vi "Vision_Left_R2.0_startup_test.vi"() -> ()   [LabVIEW 2015]
uses:
  <vilib>/vision/Pattern Matching.llb/IMAQ Curve Parameters.ctl
  <vilib>/vision/Pattern Matching.llb/IMAQ Match Range Setting.ctl
panel:
  in  "Sub - 2 File Path 2******":path=path "/home/lvuser/natinst/bin/BeaconTemplates/2_beacons_right.png"
  out "New Min Score":dbl=879.6385864257812
  out "New Low Scale":dbl=38.665856552124026
  out "New high Scale":dbl=79.77148170471192
  in  "Absolute\nMinimum Score":dbl=800.0
  in  "Absolute\nMaximum Scale":dbl=300.0
  in  "Absolute\nMinimum Scale":dbl=10.0
  in  "Score Decay \nFactor":dbl=50.0
  in  "ROI_factor(Horiztonal) (4 b)":sgl=5.0
  in  "ROI_factor(vertical) (4 b)":sgl=1.5
  in  "ROI_factor(vertical) (5 b)":sgl=2.7
  in  "ROI_factor(Horiztonal) (5 b)":sgl=4.7
  in  "ROI_factor(Horiztonal) (2 b)":sgl=1.5
  in  "ROI_factor(vertical) (2 b)":sgl=2.5
  in  "Minimum Score\nSub 2":dbl=950.0
  in  "Minimum Score\nSub 3":dbl=900.0
  in  "Minimum Score\nSub 4":dbl=850.0
  in  "Minimum Score\nNormal 5":dbl=800.0
  in  "ROBOT STATE\n(fwd, bwd, neither)":i32
  out "Scale \nCushion":dbl=20.552812576293945
  in  "Score\nCushion":dbl=150.0
  in  "Default No Lock\nSetting Values":T1={"Min Scale"=20.0, "Max Scale"=170.0, "Min Score"=800.0}
  out "Next Template":T2(ring)=enum."Normal - 5"
  in  "4 / 3\nTransition Scale":sgl=85.0
  in  "5 / 4\nTransition Scale":sgl=60.0
  in  "3 / 2\nTransition Scale":sgl=100.0
  in  "Avg Scale - Last":dbl=59.21866912841797
  in  "Avg Score - Last":dbl=954.6385864257812
  in  "Max Window\n for Avg":u8=5
  in  "Valid Treshold\nfor Lock":i16=3
  out "Current  Score":sgl=951.2561
  out "Current  Scale":sgl=59.269463
  out "Current Valid?":bool
  out "Beacon - Scales":sgl[](array[numeric])=[0.0, 59.087868, 59.67315, 57.828133, 55.61106]
  out "beacon - Scores":sgl[](array[numeric])=[0.0, 997.01117, 999.39996, 999.517, 998.72253]
  out "Beacons Found":bool[](array[boolean])=[FALSE, TRUE, TRUE, TRUE, TRUE]
  in  "Horiztonall Beacon \nCushion (pixels)":sgl=20.0
  in  "Sub - 4 - FIle Path":path=path "/home/lvuser/natinst/bin/BeaconTemplates/4_beacons_left.png"
  in  "Sub - 2 File Path":path=path "/home/lvuser/natinst/bin/BeaconTemplates/2_beacons_left.png"
  in  "Sub Beacon Template File Path - ARRAY":path[](array[path])=[path "/home/lvuser/natinst/bin/BeaconTemplates/Sub1.png", path "/home/lvuser/natinst/bin/BeaconTemplates/Sub2.png", path "/home/lvuser/natinst/bin/BeaconTemplates/Sub3.png", path "/home/lvuser/natinst/bin/BeaconTemplates/Sub4.png", path "/home/lvuser/natinst/bin/BeaconTemplates/Sub5.png"]
  in  "Sub - 3 - FIle Path":path=path "/home/lvuser/natinst/bin/BeaconTemplates/3_beacons_left.png"
  in  "Normal - 5 - File Path":path=path "/home/lvuser/natinst/bin/BeaconTemplates/5_beacons.png"
  out "Tracking Info":T3={"Tracking Coordinates"={"X"=154.8973846435547, "Y"=87.84130859375}, "Current Valid"=TRUE, "Current State - Out"=enum."Sub - 2", "Setting Values"={"Min Scale"=103.51155548095704, "Max Scale"=214.8787582397461, "Min Score"=950.0}}
  out "Current Template":T2(ring)
  in  "Initial Template":T2(ring)
  out "dT":u32=1105
  out "Avg Scale":dbl=159.2824279785156
  out "Avg Score":dbl=995.22490234375
  out "Current Search Settings":T6={"Curve Parameters"={"Extraction Mode"=1, "Edge Threshold"=150, "Edge Filter Size"=0, "Min Length"=15, "Row Search Step Size"=10, "Col Search Step Size"=10, "Max Endpoint Gap"=2, "Closed"=TRUE, "Subpixel"=TRUE}, "Match Mode"={"Rotation"=FALSE, "Scale"=TRUE, "Occlusion"=TRUE, "Reserved"=FALSE, "Reserved"=FALSE, "Reserved"=FALSE}, "Range Settings"=[{"Match Constraints"=0, "Min"=-2.0, "Max"=2.0}, {"Match Constraints"=1, "Min"=103.59702987670897, "Max"=214.96782608032225}, {"Match Constraints"=2, "Min"=0.0, "Max"=20.0}], "Number of Matches"=1, "Minimum Match Score"=950.0, "SubPixel Accuracy"=TRUE, "Adv. Geometric Match Options 2"=[{"Setup Data Item"=20, "Item Value"=0.0}, {"Setup Data Item"=22, "Item Value"=1.0}]} {"Curve Parameters"."Extraction Mode" items=["Normal", "Uniform Regions"]; "Curve Parameters"."Edge Filter Size" items=["Fine", "Normal", "Contour Tracing"]; "Curve Parameters"."Max Endpoint Gap" min=0; "Curve Parameters"."Col Search Step Size" min=1 max=255 step=1; "Curve Parameters"."Row Search Step Size" min=1 max=255 step=1; "Curve Parameters"."Min Length" min=0; "Curve Parameters"."Edge Threshold" min=1 max=350 step=1; "Range Settings"."Max" format="%.2f"; "Range Settings"."Min" format="%.2f"; "Range Settings"."Match Constraints" items=["Rotation Angle (degrees)", "Scale Factor (%)", "Occlusion (%)"]}
  out "Valid Scale History":dbl[](array[numeric])=[159.54193115234375, 159.0799560546875, 159.38912963867188, 159.05020141601562, 159.35092163085938, 159.10557556152344, 159.3151092529297, 159.3177947998047, 159.0937957763672, 159.64999389648438, 159.23023986816406, 159.07296752929688, 159.37905883789062, 156.36964416503906, 151.1900634765625, 132.892578125, 119.50423431396484, 108.0020523071289, 99.8529052734375, 93.15778350830078] format="%#_13g"
  out "Valid Score History":dbl[](array[numeric])=[995.82177734375, 997.0046997070312, 997.0046997070312, 997.0046997070312, 989.2886352539062, 997.0046997070312, 997.0046997070312, 996.4745483398438, 996.4745483398438, 995.4120483398438, 996.692138671875, 996.692138671875, 996.692138671875, 996.337890625, 998.2847290039062, 996.9906616210938, 1000.0, 999.7824096679688, 999.7824096679688, 999.7824096679688] format="%#_13g"
  out "Valid Beacon History - in":bool[](array[boolean])=[TRUE, TRUE, TRUE, TRUE, TRUE, TRUE, TRUE, TRUE, TRUE, TRUE, TRUE, TRUE, TRUE, TRUE, TRUE, TRUE, TRUE, TRUE, TRUE, TRUE]
  out "Startup Flag":bool
  out "Lock Status":bool
  out "Y Coordinates":sgl[](array[numeric])=[100.60873, 0.0, 0.0, 0.0, 0.0]
  out "X Coordinates":sgl[](array[numeric])=[108.138504, 0.0, 0.0, 0.0, 0.0]
  out "Right Image out":T7(plugin-control)
  in  "History Size":i32=20
  in  "INITIAL Search Settings":T6={"Curve Parameters"={"Extraction Mode"=1, "Edge Threshold"=150, "Edge Filter Size"=0, "Min Length"=15, "Row Search Step Size"=10, "Col Search Step Size"=10, "Max Endpoint Gap"=2, "Closed"=TRUE, "Subpixel"=TRUE}, "Match Mode"={"Rotation"=FALSE, "Scale"=TRUE, "Occlusion"=TRUE, "Reserved"=FALSE, "Reserved"=FALSE, "Reserved"=FALSE}, "Range Settings"=[{"Match Constraints"=0, "Min"=-2.0, "Max"=2.0}, {"Match Constraints"=1, "Min"=90.0, "Max"=150.0}, {"Match Constraints"=2, "Min"=0.0, "Max"=20.0}], "Number of Matches"=1, "Minimum Match Score"=900.0, "SubPixel Accuracy"=TRUE, "Adv. Geometric Match Options 2"=[{"Setup Data Item"=20, "Item Value"=0.0}, {"Setup Data Item"=22, "Item Value"=1.0}]} {"Curve Parameters"."Extraction Mode" items=["Normal", "Uniform Regions"]; "Curve Parameters"."Edge Filter Size" items=["Fine", "Normal", "Contour Tracing"]; "Curve Parameters"."Max Endpoint Gap" min=0; "Curve Parameters"."Col Search Step Size" min=1 max=255 step=1; "Curve Parameters"."Row Search Step Size" min=1 max=255 step=1; "Curve Parameters"."Min Length" min=0; "Curve Parameters"."Edge Threshold" min=1 max=350 step=1; "Range Settings"."Max" format="%.2f"; "Range Settings"."Min" format="%.2f"; "Range Settings"."Match Constraints" items=["Rotation Angle (degrees)", "Scale Factor (%)", "Occlusion (%)"]; "Adv. Geometric Match Options 2"."Setup Data Item" items=["Curve Extraction Mode", "Curve Edge Threshold", "Curve Edge Filter Size", "Min Curve Length", "Curve Row Search Step Size", "Curve Col Search Step Size", "Curve Max Endpoint Gap", "Extract Closed Curves", "Enable Subpixel Curve Extraction", "Enable Correlation Score", "Enable Subpixel Accuracy", "Subpixel Iterations", "Subpixel Tolerance", "Initial Match List Length", "Enable Target Template Curve Score", "Min Match Separation Distance", "Min Match Separation Angle", "Min Match Separation Scale", "Max Match Overlap", "Enable Coarse Result", "Enable Calibration Support", "Enable Contrast Reversal", "Search Strategy", "Refinement Match Factor", "Subpixel Match Factor"]}
  # "TEMPLATE FILE PATHS"
  # "Current Match Values"
  # "Range"
  # "Range"
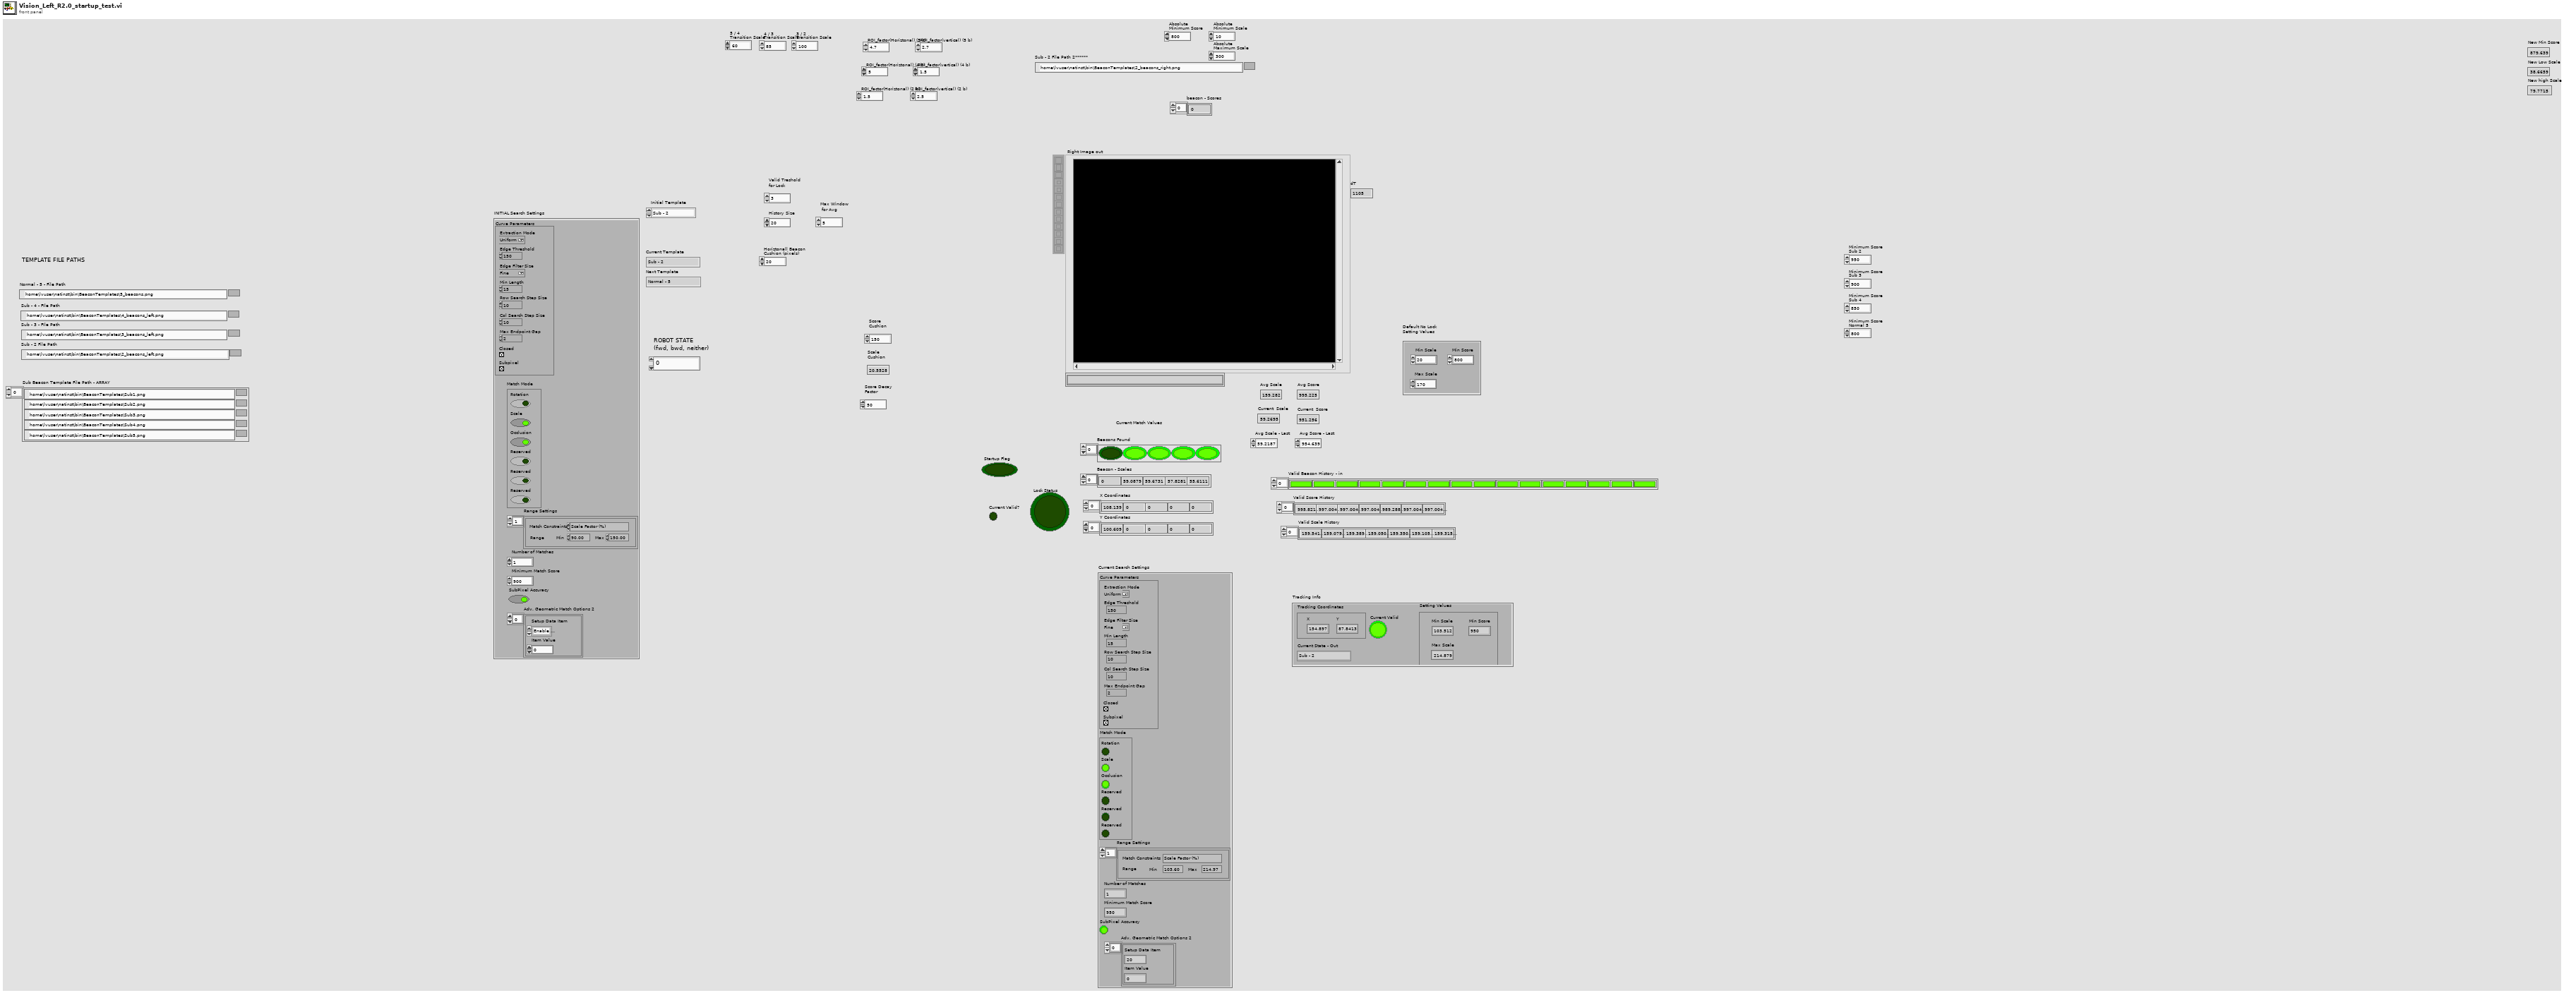
[diagram p1: front panel]
types:
  T1 = cluster{"Min Scale":dbl, "Max Scale":dbl, "Min Score":dbl}
  T2 = enum16{"Sub - 2", "Sub - 3", "Sub - 4", "Normal - 5"}
  T3 = cluster{"Tracking Coordinates":cluster{"X":dbl, "Y":dbl}, "Current Valid":bool, "Current State - Out":enum16{"Sub - 2", "Sub - 3", "Sub - 4", "Normal - 5"}, "Setting Values":cluster{"Min Scale":dbl, "Max Scale":dbl, "Min Score":dbl}}
  T4 = typedef "IMAQ Curve Parameters.ctl" = cluster{"Extraction Mode":u32, "Edge Threshold":i32, "Edge Filter Size":u32, "Min Length":i32, "Row Search Step Size":i32, "Col Search Step Size":i32, "Max Endpoint Gap":i32, "Closed":bool, "Subpixel":bool}
  T5 = typedef "IMAQ Match Range Setting.ctl" = cluster{"Match Constraints":u32, "Min":dbl, "Max":dbl}
  T6 = cluster{"Curve Parameters":T4, "Match Mode":cluster{"Rotation":bool, "Scale":bool, "Occlusion":bool, "Reserved":bool, "Reserved":bool, "Reserved":bool}, "Range Settings":T5[], "Number of Matches":i32, "Minimum Match Score":sgl, "SubPixel Accuracy":bool, "Adv. Geometric Match Options 2":cluster{"Setup Data Item":u16, "Item Value":dbl}[]}
  T7 = typedef "IMAQ Image.ctl" = refnum<image>
  T8 = typedef "Image Type" = u32
  T9 = typedef "ROI Descriptor" = cluster{"Global Rectangle":i32[], "Contours":cluster{"ID":enum32{"External", "Internal"}, "Type":u32, "Coordinates":i32[]}[]}
  T10 = typedef "IMAQ GM Match Report.ctl" = cluster{"Position":cluster{"x":sgl, "y":sgl}, "Angle":sgl, "Scale":sgl, "Score":sgl, "Bounding Box":cluster{"x":sgl, "y":sgl}[], "Contrast Reversed":bool, "Occlusion %":sgl, "Template Target Curve Score":sgl, "Target Template Curve Score":sgl, "Correlation Score":sgl}
  T11 = cluster{"Matches (Geometric Matching 1)[0]":T10, "Matches (Geometric Matching 1)[1]":T10, "Matches (Geometric Matching 1)[2]":T10, "Matches (Geometric Matching 1)[3]":T10, "Matches (Geometric Matching 1)[4]":T10, "Matches (Geometric Matching 1)[5]":T10, "Matches (Geometric Matching 1)[6]":T10, "Matches (Geometric Matching 1)[7]":T10, "Matches (Geometric Matching 1)[8]":T10}
  T12 = cluster{"Bounding Box[0]":cluster{"x":sgl, "y":sgl}, "Bounding Box[1]":cluster{"x":sgl, "y":sgl}, "Bounding Box[2]":cluster{"x":sgl, "y":sgl}, "Bounding Box[3]":cluster{"x":sgl, "y":sgl}, "Bounding Box[4]":cluster{"x":sgl, "y":sgl}, "Bounding Box[5]":cluster{"x":sgl, "y":sgl}, "Bounding Box[6]":cluster{"x":sgl, "y":sgl}, "Bounding Box[7]":cluster{"x":sgl, "y":sgl}, "Bounding Box[8]":cluster{"x":sgl, "y":sgl}}
  T13 = typedef "IMAQ Rectangle" = cluster{"Left":i32, "Top":i32, "Right":i32, "Bottom":i32, "Rotation":dbl}
  T14 = cluster{"Minimum Score\nNormal 5":dbl, "Min":dbl, "Max":dbl}
  T15 = cluster{"Position":cluster{"x":dbl, "y":dbl}, bool, "Next Template":enum16{"Sub - 2", "Sub - 3", "Sub - 4", "Normal - 5"}, cluster{"Minimum Score\nNormal 5":dbl, "Min":dbl, "Max":dbl}}
  T16 = cluster{"Position":cluster{"x":dbl, "y":dbl}, bool, "Current Template":enum16{"Sub - 2", "Sub - 3", "Sub - 4", "Normal - 5"}, cluster{"Minimum Score\nNormal 5":dbl, "Min":dbl, "Max":dbl}}
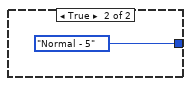
[diagram p3: hidden frame]
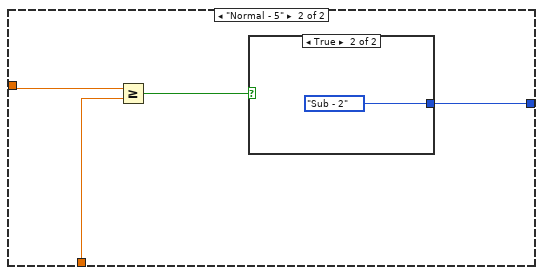
[diagram p4: hidden frame]
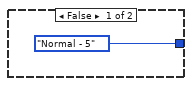
[diagram p5: hidden frame]
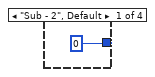
[diagram p7: hidden frame]
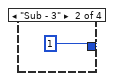
[diagram p8: hidden frame]
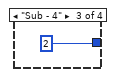
[diagram p9: hidden frame]
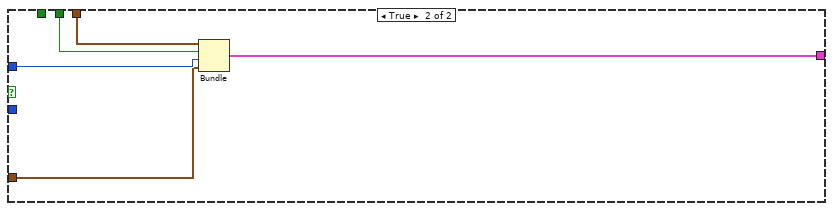
[diagram p10: hidden frame]
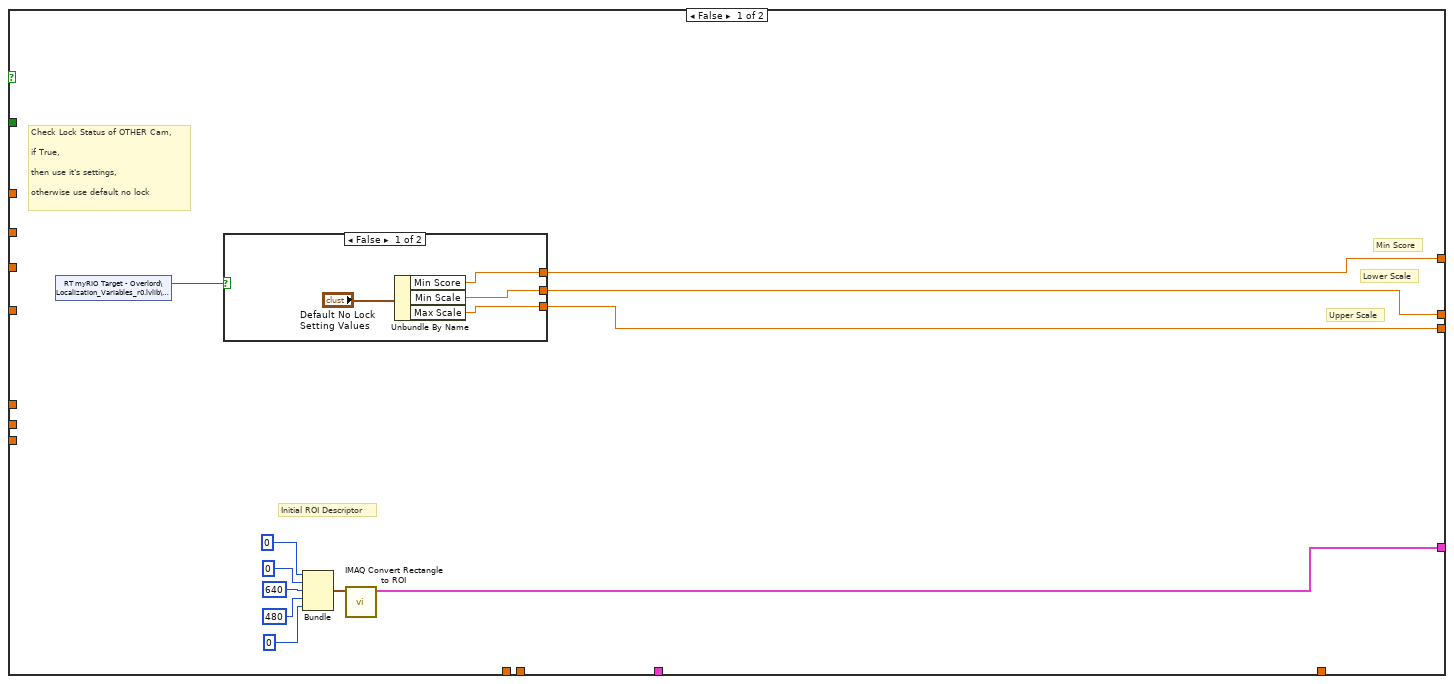
[diagram p13: hidden frame]
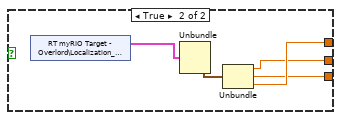
[diagram p14: hidden frame]
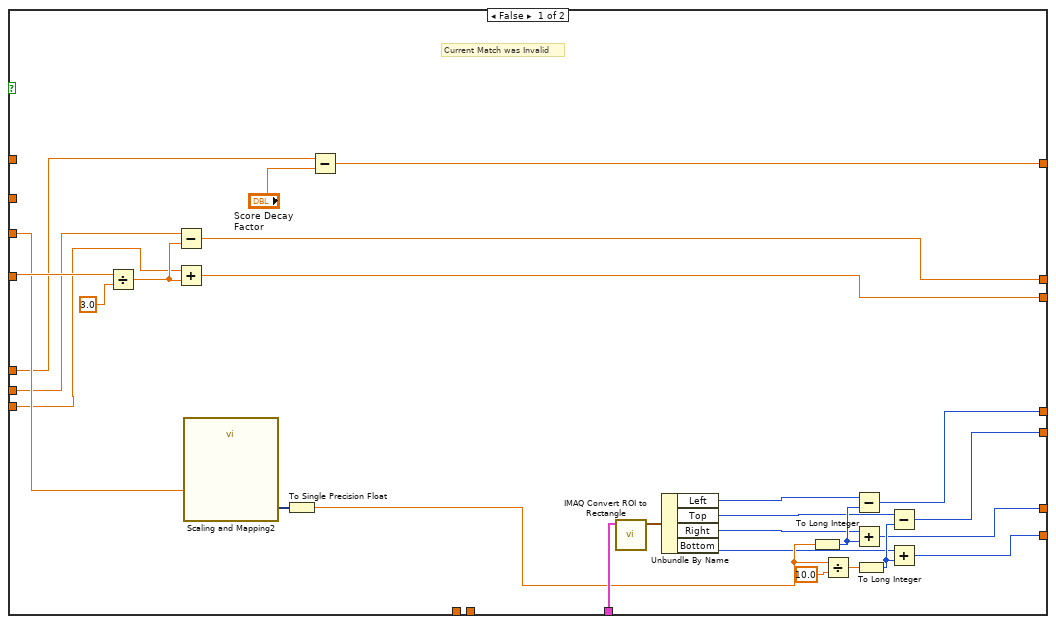
[diagram p15: hidden frame]
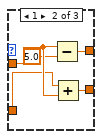
[diagram p16: hidden frame]
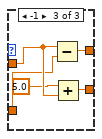
[diagram p17: hidden frame]
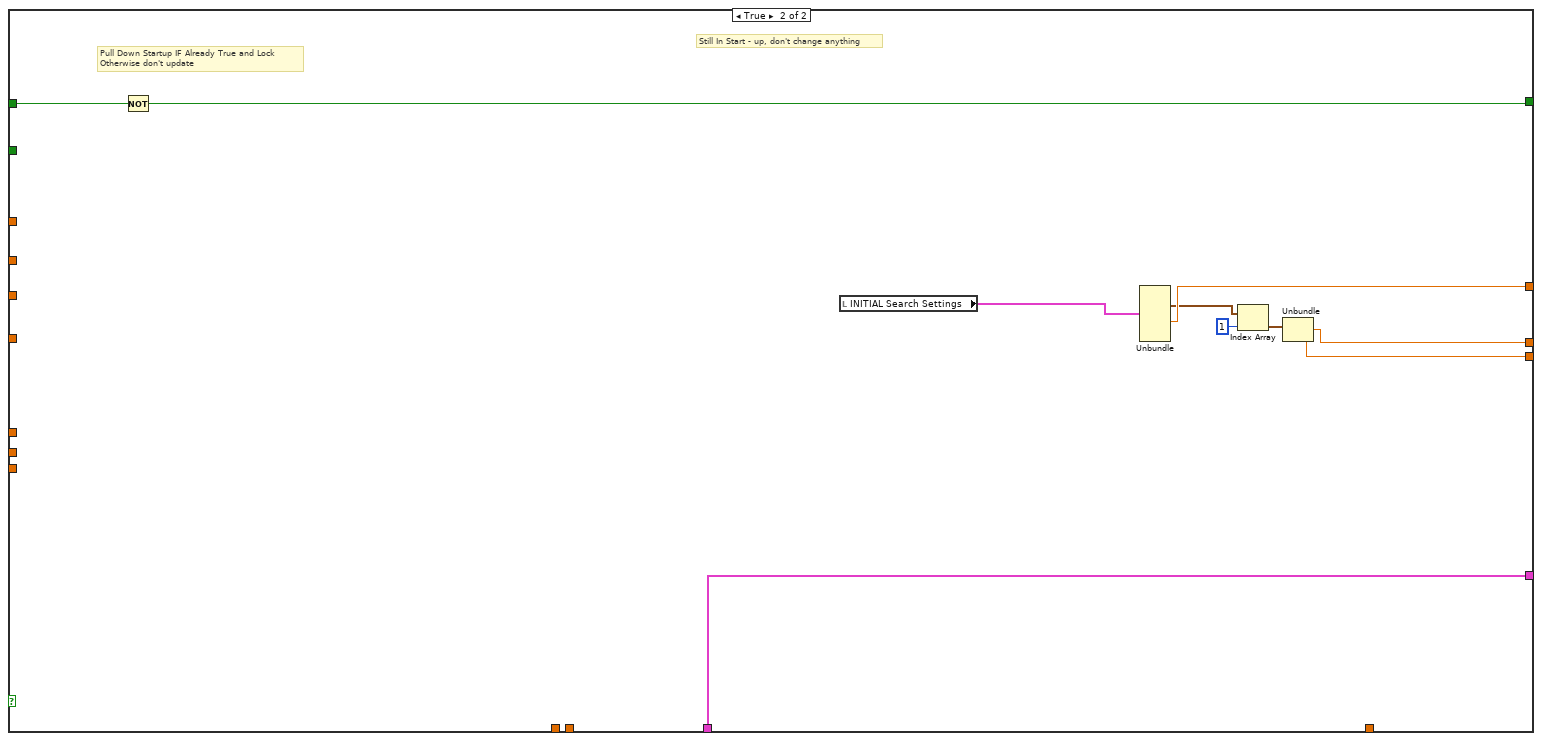
[diagram p18: hidden frame]
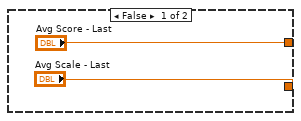
[diagram p19: hidden frame]
diagram:
  n1 = flat-sequence {
    tunnel: [w24] -> w12
    tunnel: ["INITIAL Search Settings"] -> w11
    tunnel: ["Initial Template"] -> w10
    tunnel: [TRUE] -> w9
    tunnel: [w21] -> w8
    tunnel: [w20] -> w7
    tunnel: [w19] -> w6
    tunnel: [w18] -> w5
    tunnel: [w17] -> w4
    tunnel: ["History Size"] -> w3
    tunnel: [750.0] -> w2
    tunnel: [100.0] -> w1
    tunnel: w12 -> [w46]
    tunnel: w11 -> [w45]
    tunnel: w10 -> [w44]
    tunnel: w9 -> [w43]
    tunnel: w8 -> [w39]
    tunnel: w7 -> [w36]
    tunnel: w6 -> [w42]
    tunnel: w5 -> [w41]
    tunnel: w4 -> [w40]
    tunnel: w3 -> [w38]
    tunnel: w2 -> [_]
    tunnel: w1 -> [_]
    frame #0 {
      w31 = T8 0 items=["Grayscale (U8)", "Grayscale (I16)", "Grayscale (SGL)", "Complex (CSG)", "RGB (U32)", "HSL (U32)", "RGB (U64)", "Grayscale (U16)"] ("Image Type")
      # "avg start scale"
      # "Score History"
      # "Scale History"
      # "Valid Match History\n(main beacon)"
      # "Template State"
      # "Search Parameters"
      # "StartUp = True"
      # "Initial ROI Descriptor"
      # "INITIALIZE"
      n2 = Bundle(0, 0, 640, 480, 0) -> (w30:cluster{i32, i32, i32, i32, i32})  [unwired: 1 in]
      n3 = call "IMAQ Convert Rectangle to ROI"("Rectangle"=w30) -> ("ROI Descriptor"=w24:T9)  [unwired: 8 in, 1 out]
      n4 = call "IMAQ Create"("Image Name"="Left_Image", "Image Type"=w31) -> ("New Image"=w21:T7, "error out"=w20:errorcluster)  [unwired: 3 in]
      n5 = Initialize Array(FALSE, "History Size") -> (w19:bool[])
      n6 = Initialize Array(0.0, "History Size") -> (w17:dbl[])
      n7 = Initialize Array(0.0, "History Size") -> (w18:dbl[])
    }
    frame #1 {
      # "Avg Scale"
      # "Avg Score"
      # "Score History"
      # "Scale History"
      # "Valid Match History\n(main beacon)"
      # "Sub Beacon Search Array"
      # "StartUp = True"
      # "Template State"
      # "Search Parameters"
      # "ROI"
      n8 = call "Tick Count"() -> ("Tick Count(mSec)"=w37:u32)
      n9 = while {
        shift-right: [w58] -> _
        shift-left: w46 -> [w65]
        shift-right: [w59] -> _
        shift-left: w45 -> [w66]
        shift-right: [w56] -> _
        shift-left: w44 -> [w74]
        shift-right: [w62] -> _
        shift-left: w43 -> [w64]
        shift-right: [w51] -> _
        shift-left: w42 -> [w52]
        shift-right: [w49] -> _
        shift-left: w41 -> [w50]
        shift-right: [w47] -> _
        shift-left: w40 -> [w48]
        shift-right: [w54] -> _
        shift-left: w39 -> [w67]
        tunnel: w38 -> [w72]
        shift-right: [w70] -> _
        shift-left: w37 -> [w71]
        tunnel: w36 -> [w53]
        stop <- FALSE stop-if-true
        n10 = call "Tick Count2"() -> ("Tick Count(mSec)"=w70:u32)
        n11 = Subtract(x=w70, y=w71) -> (x-y=→"dT":u32)
        n12 = flat-sequence {
          tunnel: [w81] -> w75
          tunnel: [w80] -> w73
          tunnel: [w79] -> w61
          tunnel: [w78] -> w68
          tunnel: w67 -> [w78]
          tunnel: [w78] -> w54
          tunnel: w53 -> [w77]
          tunnel: w75 -> [w191]
          tunnel: w74 -> [w87]
          tunnel: w73 -> [w93]
          tunnel: w52 -> [w170]
          tunnel: w50 -> [w169]
          tunnel: w48 -> [w168]
          tunnel: w72 -> [_]
          tunnel: w68 -> [w185]
          tunnel: w66 -> [w113]
          tunnel: w65 -> [w136]
          tunnel: w64 -> [w153]
          tunnel: [w112] -> w63
          tunnel: [w107] -> w62
          tunnel: w61 -> [w96]
          tunnel: [w96] -> w60
          tunnel: [w95] -> w57
          tunnel: [w94] -> w55
          tunnel: [w90] -> w51
          tunnel: [w89] -> w49
          tunnel: [w88] -> w47
          tunnel: w63 -> [w582]
          tunnel: w60 -> [w583]
          tunnel: [w582] -> w59
          tunnel: [w581] -> w58
          tunnel: w57 -> [w581]
          tunnel: [w580] -> w56
          tunnel: w55 -> [w580]
          frame #0 {
            # "Aquire Image"
            n13 = shared-variable "RT myRIO Target - Overlord\\Localization_Variables_r0.lvlib\\Left Servo Angle_Current"() -> (w79:dbl)  [unwired: 1 in, 1 out]
            n14 = call "Camera Acquisition"("error in"=w77) -> ("Image Out"=w81:T7, "error out"=w80:errorcluster)  [unwired: 24 in, 1 out]
          }
          frame #1 {
            w116 = u32 1 ("index")
            # "Current Template"
            # "Check if Next Template == Current TEmplate"
            # "Update Tracking Coordinates"
            # "Next Settings"
            # "Current Settings"
            # "Current Min\n& Max Scale"
            # "Scale"
            # "Min Score"
            # "Lower Scale"
            # "Upper Scale"
            # "Min Score out"
            # "Choose ROI Factor based on Next State"
            # "Avg Scale"
            # "Avg Score"
            # "StartUp Flag"
            # "Current Valid"
            # "image Lock"
            # "Update Search Settings"
            # "Image Lock?"
            # "Update Template"
            # "Score History"
            # "Min Required to use avarage"
            # "Scale History"
            # "History Size"
            # "Calculate Average Score/Scale"
            # "****# of previous in history that must be true\nin order for position to be considered \"locked\""
            # "Scale History"
            # "Score History"
            # "Valid History"
            # "Update History Data"
            # "1 Match FOund?"
            # "# of Sub Beacons"
            # "Sub Beacons to Search For"
            # "# Sub Beacons to Find in\norder to be valid"
            # "Template Filepath"
            # "Select Current Template Config"
            # "Pattern Match to Current Template"
            # "Apply FIltering"
            n15 = call "Camera - Filtering"("Image In"=w191, "Image Dst"=w185, "error in"=w93) -> ("Image Out"=w186:T7, "error out"=w92:errorcluster)  [unwired: 23 in]
            n16 = case shown="\"Normal - 5\"" w87 {
              tunnel: "Normal - 5 - File Path" -> [_ _ _ w579]
              tunnel: "Sub - 4 - FIle Path" -> [_ _ w574 _]
              tunnel: "Sub - 3 - FIle Path" -> [_ w568 _ _]
              tunnel: "Sub - 2 File Path" -> [w562 _ _ _]
              tunnel: [w562 w568 w574 w579] -> w184
              tunnel: [1 2 3 4] -> w172
              tunnel: [w560 w565 w571 w576] -> w177
              tunnel: [sgl 2.0 sgl 3.0 sgl 4.0 sgl 5.0] -> w178
              tunnel: "Sub - 2 File Path 2******" -> [_ _ _ _]
              frame "Sub - 2", Default {
                w558 = FALSE
                w559 = TRUE
                n17 = Build Array(w559, w559, w558, w558, w558) -> (w560:bool[])
              }
              frame "Sub - 3" {
                w564 = FALSE
                w566 = TRUE
                n18 = Build Array(w566, w566, w566, w564, w564) -> (w565:bool[])
              }
              frame "Sub - 4" {
                w572 = TRUE
                n19 = Build Array(w572, w572, w572, w572, FALSE) -> (w571:bool[])
              }
              frame "Normal - 5" {
                (unwired) FALSE
                w577 = TRUE
                n20 = Build Array(w577, w577, w577, w577, w577) -> (w576:bool[])
              }
            }
            n21 = call "Geometric Pattern Matching"("Image In"=w186, "Image Dst"=w185, "ROI Descriptor (Geometric Matching 1)"=w136, "Settings (Geometric Matching 1)"=w113, "Template File Path (Geometric Matching 1)"=w184, "error in"=w92) -> ("Image Out"=w179:T7, "Matches (Geometric Matching 1)"=w180:T10[], "Number of Matches (Geometric Matching 1)"=w183:i32, "error out"=w176:errorcluster)  [unwired: 18 in]
            n22 = Equal?(x=w183, y=1) -> (x = y?=w181:bool)
            n23 = case shown="True" w181 {
              tunnel: w180 -> [_ w505]
              tunnel: w179 -> [w461 w484]
              tunnel: w178 -> [_ w499]
              tunnel: w177 -> [_ w486]
              tunnel: w176 -> [_ w483]
              tunnel: w113 -> [_ w481]
              tunnel: [w466 w479] -> w100
              tunnel: [w465 w478] -> w99
              tunnel: [w465 w477] -> w98
              tunnel: [w465 w476] -> w97
              tunnel: [w465 w475] -> w173
              tunnel: [w464 w474] -> w167
              tunnel: [w464 w473] -> w166
              tunnel: [w461 w472] -> w111
              tunnel: [w462 w471] -> w108
              frame False {
                w463 = 0.0
                w464 = sgl 0.0 ("Scale")
                n24 = Bundle(w463, w463) -> (w462:cluster{dbl, dbl})  [unwired: 1 in]
                n25 = Initialize Array(FALSE, 5 ("dimension size")) -> (w466:bool[])
                n26 = Initialize Array(0.0, 5 ("dimension size")) -> (w465:dbl[])
              }
              frame True {
                # "Build ROI for Individual Beacons Based on Main Bounding Box"
                # "Starting X Lower Bound"
                # "Beacons to Search For"
                # "Length of\nIndividual Beacon ROI"
                # "Length of Bounding Box"
                # "Draw Bounding Box on Display Image"
                n27 = Array To Cluster(array=w505) -> (cluster=w506:T11)
                n28 = Unbundle By Name(w506) -> ("Matches (Geometric Matching 1)[0].Position"=w471:cluster{"x":sgl, "y":sgl}, "Matches (Geometric Matching 1)[0].Bounding Box"=w503:cluster{"x":sgl, "y":sgl}[], "Matches (Geometric Matching 1)[0].Scale"=w474:sgl, "Matches (Geometric Matching 1)[0].Score"=w473:sgl)
                n29 = Array To Cluster(array=w503) -> (cluster=w504:T12)
                n30 = Unbundle By Name(w504) -> ("Bounding Box[0].x"=w497:sgl, "Bounding Box[0].y"=w493:sgl, "Bounding Box[2].x"=w500:sgl, "Bounding Box[2].y"=w492:sgl)
                n31 = Bundle("x"=w497, "y"=w493, "x"=w500, "y"=w492) -> (w502:cluster{"x":sgl, "y":sgl, "x":sgl, "y":sgl})  [unwired: 1 in]
                n32 = call "IMAQ Overlay Rectangle"("Rectangle"=w502, "Image"=w484) -> ("Image Out"=w480:T7)  [unwired: 8 in, 1 out]
                n33 = Subtract(x=w500, y=w497) -> (x-y=w501:sgl)
                n34 = Divide(x=w501, y=w499) -> (x/y=w498:sgl)
                n35 = Multiply(x="Horiztonall Beacon \nCushion (pixels)", y=w474) -> (x*y=w494:sgl)
                n36 = Divide(x=w494, y=sgl 100.0) -> (x/y=w489:sgl)
                n37 = Subtract(x=w493, y=w489) -> (x-y=w491:sgl)
                n38 = Add(x=w492, y=w489) -> (x+y=w490:sgl)
                n39 = for {
                  N: 5 -> [_]
                  tunnel: w486 -> [w552] mode=indexing
                  shift-right: [w546] -> _
                  shift-left: w497 -> [w551]
                  tunnel: w498 -> [w550]
                  tunnel: w491 -> [w543]
                  tunnel: w490 -> [w542]
                  tunnel: [w549] -> w485 mode=indexing
                  tunnel: w489 -> [w544]
                  # "Divide Bounding Box"
                  # "Upper Bound of Current is\nLower Bound for Next"
                  n40 = case shown="True" w552 {
                    tunnel: w551 -> [w553 w554]
                    tunnel: w550 -> [_ w556]
                    tunnel: [w553 w555] -> w546
                    tunnel: [w553 w554] -> w548
                    frame False {
                      # "Don't Care"
                    }
                    frame True {
                      # "X Lower Bound"
                      n41 = Add(x=w554, y=w556) -> (x+y=w555:sgl)
                    }
                  }
                  n42 = Subtract(x=w548, y=w544) -> (x-y=w547:sgl)
                  n43 = Add(x=w546, y=w544) -> (x+y=w545:sgl)
                  n44 = call "Bound_RO_R_R0I.vi"("Bottom Right - Y"=w542, "Right - X"=w545, "Top Left - Y"=w543, "Top  Left - x"=w547) -> ("ROI Descriptor"=w549:T9)  [unwired: 7 in]
                }
                n45 = for {
                  N: 5 -> [_]
                  tunnel: w484 -> [w519]
                  tunnel: w483 -> [w518]
                  tunnel: w485 -> [w511] mode=indexing
                  tunnel: "Sub Beacon Template File Path - ARRAY" -> [w517] mode=indexing
                  tunnel: [w516] -> w478 mode=indexing
                  tunnel: [w515] -> w477 mode=indexing
                  tunnel: [w514] -> w479 mode=indexing
                  tunnel: w486 -> [w513] mode=indexing
                  tunnel: w481 -> [w512]
                  shift-right: [w509] -> w472
                  shift-left: w480 -> [w510]
                  tunnel: [w508] -> w476 mode=indexing
                  tunnel: [w507] -> w475 mode=indexing
                  n46 = case shown="True" w513 {
                    tunnel: w519 -> [_ w534]
                    tunnel: w518 -> [_ w533]
                    tunnel: w511 -> [_ w532]
                    tunnel: w517 -> [_ w531]
                    tunnel: [w520 w527] -> w516
                    tunnel: [w520 w526] -> w515
                    tunnel: [FALSE w525] -> w514
                    tunnel: w512 -> [_ w524]
                    tunnel: [w520 w523] -> w508
                    tunnel: [w520 w522] -> w507
                    frame False {
                      w520 = sgl 0.0 ("x")
                    }
                    frame True {
                      n47 = call "Sub Beacon Pattern Match"("Image In"=w534, "ROI Descriptor (Geometric Matching 1)"=w532, "Settings (Geometric Matching 1)"=w524, "Template File Path (Geometric Matching 1)"=w531, "error in"=w533) -> ("Matches (Geometric Matching 1)"=w528:T10[], "Number of Matches (Geometric Matching 1)"=w529:i32)  [unwired: 19 in, 2 out]
                      n48 = Equal?(x=w529, y=1) -> (x = y?=w525:bool)
                      n49 = case shown="True" w525 {
                        tunnel: w528 -> [_ w540]
                        tunnel: [w535 w539] -> w527
                        tunnel: [w535 w538] -> w526
                        tunnel: [w535 w537] -> w523
                        tunnel: [w535 w536] -> w522
                        frame False {
                          w535 = sgl 0.0 ("x")
                        }
                        frame True {
                          n50 = Array To Cluster(array=w540) -> (cluster=w541:T11)
                          n51 = Unbundle By Name(w541) -> ("Matches (Geometric Matching 1)[0].Position.x"=w539:sgl, "Matches (Geometric Matching 1)[0].Position.y"=w538:sgl, "Matches (Geometric Matching 1)[0].Scale"=w537:sgl, "Matches (Geometric Matching 1)[0].Score"=w536:sgl)
                        }
                      }
                    }
                  }
                  n52 = call "IMAQ Overlay ROI"("ROI Descriptor"=w511, "Image"=w510) -> ("Image Out"=w509:T7)  [unwired: 8 in, 1 out]
                }
              }
            }
            "Beacons Found" <- w100
            "X Coordinates" <- w99
            "Y Coordinates" <- w98
            "Beacon - Scales" <- w97
            "beacon - Scores" <- w173
            "Current  Scale" <- w167
            "Current  Score" <- w166
            n53 = shared-variable "RT myRIO Target - Overlord\\Localization_Variables_r0.lvlib\\LEFT_BEACON_BOOL_array"(w100) -> ()  [unwired: 1 in, 1 out]
            n54 = shared-variable "RT myRIO Target - Overlord\\Localization_Variables_r0.lvlib\\LEFT_BEACON_X_array"(w99) -> ()  [unwired: 1 in, 1 out]
            n55 = shared-variable "RT myRIO Target - Overlord\\Localization_Variables_r0.lvlib\\LEFT_BEACON_Y_array"(w98) -> ()  [unwired: 1 in, 1 out]
            n56 = shared-variable "RT myRIO Target - Overlord\\Localization_Variables_r0.lvlib\\LEFT_BEACON_Scales"(w97) -> ()  [unwired: 1 in, 1 out]
            n57 = Boolean To (0,1)(Boolean=w100) -> (0, 1=w175:i16[])
            n58 = Add Array Elements(numeric array=w175) -> (sum=w174:i16)
            n59 = Greater Or Equal?(x=w174, y=w172) -> (x >= y?=w91:bool)
            "Current Valid?" <- w91
            n60 = local read "History Size"() -> (w158:i32)
            n61 = Decrement(x=w158) -> (x-1=w171:i32)
            n62 = for {
              N: w158 -> [_]
              shift-right: [w439] -> w90
              shift-left: w170 -> [w427]
              tunnel: w171 -> [w435]
              shift-right: [w432] -> w89
              shift-left: w169 -> [w434]
              shift-right: [w431] -> w88
              shift-left: w168 -> [w433]
              tunnel: w167 -> [w430]
              tunnel: w166 -> [w429]
              tunnel: w91 -> [w428]
              i -> [w438]
              # "Reverse Index"
              n63 = Subtract(x=w435, y=w438) -> (x-y=w436:i32)
              n64 = Equal To 0?(x=w436) -> (x = 0?=w437:bool)
              n65 = case shown="True" w437 {
                tunnel: w436 -> [w440 w459]
                tunnel: w427 -> [w450 w452]
                tunnel: [w448 w451] -> w439
                tunnel: w428 -> [_ w460]
                tunnel: w434 -> [w445 w458]
                tunnel: w433 -> [w444 w457]
                tunnel: [w443 w455] -> w432
                tunnel: [w442 w456] -> w431
                tunnel: w430 -> [_ w454]
                tunnel: w429 -> [_ w453]
                frame False {
                  # "Shift Old"
                  n66 = Decrement(x=w440) -> (x-1=w441:i32)
                  n67 = Index Array(array=w450, index=w441) -> (element=w449:bool)
                  n68 = Index Array(array=w445, index=w441) -> (element=w447:dbl)
                  n69 = Index Array(array=w444, index=w441) -> (element=w446:dbl)
                  n70 = Replace Array Subset(array=w450, new element=w449, index=w440) -> (w448:bool[])
                  n71 = Replace Array Subset(array=w445, new element=w447, index=w440) -> (w443:dbl[])
                  n72 = Replace Array Subset(array=w444, new element=w446, index=w440) -> (w442:dbl[])
                }
                frame True {
                  # "Score"
                  # "Scale"
                  # "Valid"
                  # "insert New"
                  n73 = Replace Array Subset(array=w458, new element=w454, index=w459) -> (w455:dbl[])
                  n74 = Replace Array Subset(array=w457, new element=w453, index=w459) -> (w456:dbl[])
                  n75 = Replace Array Subset(array=w452, new element=w460, index=w459) -> (w451:bool[])
                }
              }
            }
            n76 = Boolean To (0,1)(Boolean=w90) -> (0, 1=w164:i16[])
            n77 = Add Array Elements(numeric array=w164) -> (sum=w163:i16)
            n78 = Greater Or Equal?(x=w163, y="Valid Treshold\nfor Lock") -> (x >= y?=w85:bool)
            "Lock Status" <- w85
            n79 = shared-variable "RT myRIO Target - Overlord\\Localization_Variables_r0.lvlib\\Image Lock - L"(w85) -> ()  [unwired: 1 in, 1 out]
            n80 = Initialize Array(u8 0, "Max Window\n for Avg") -> (w161:u8[])
            n81 = while {
              shift-right: [w410] -> w157
              shift-left: w161 -> [w412]
              tunnel: w90 -> [w418] mode=indexing
              shift-right: [w416] -> w154
              shift-left: u8 0 -> [w419]
              tunnel: w158 -> [w417]
              tunnel: "Max Window\n for Avg" -> [w409]
              i -> [w411]
              stop <- w413 stop-if-true
              # "Grab Last 'X' Valid Indexes"
              n82 = case shown="True" w418 {
                tunnel: w419 -> [w421 w423]
                tunnel: [w421 w426] -> w416
                tunnel: w412 -> [w420 w425]
                tunnel: w411 -> [_ w424]
                tunnel: [w420 w422] -> w410
                frame False {
                }
                frame True {
                  # "Update Index\nto use"
                  # "Increment\nValid Count"
                  n83 = Replace Array Subset(array=w425, new element=w424, index=w423) -> (w422:u8[])
                  n84 = Increment(x=w423) -> (x+1=w426:u8)
                }
              }
              n85 = Greater?(x=w411, y=w417) -> (0:w414:bool)
              n86 = Greater Or Equal?(x=w416, y=w409) -> (x >= y?=w415:bool)
              n87 = Or(x=w415, y=w414) -> (x .or. y?=w413:bool)
            }
            n88 = Greater Or Equal?(x=w154, y=u8 2) -> (x >= y?=w155:bool)
            n89 = case shown="True" w155 {
              tunnel: w154 -> [_ w393]
              tunnel: w157 -> [_ w399]
              tunnel: w89 -> [_ w398]
              tunnel: w88 -> [_ w397]
              tunnel: ["Avg Score - Last" w391] -> w84
              tunnel: ["Avg Scale - Last" w390] -> w149
              frame False {
              }
              frame True {
                w396 = 0.0
                n90 = for {
                  N: w393 -> [_]
                  tunnel: w399 -> [w406] mode=indexing
                  tunnel: w398 -> [w408]
                  tunnel: w397 -> [w407]
                  shift-right: [w404] -> w395
                  shift-left: w396 -> [w402]
                  shift-right: [w405] -> w394
                  shift-left: w396 -> [w401]
                  # "Fetch Last Valid Values"
                  n91 = Index Array(array=w408, index=w406) -> (element=w403:dbl)
                  n92 = Index Array(array=w407, index=w406) -> (element=w400:dbl)
                  n93 = Add(x=w403, y=w402) -> (x+y=w404:dbl)
                  n94 = Add(x=w400, y=w401) -> (x+y=w405:dbl)
                }
                n95 = To Double Precision Float(number=w393) -> (double precision float=w392:dbl)
                n96 = Divide(x=w395, y=w392) -> (x/y=w391:dbl)
                n97 = Divide(x=w394, y=w392) -> (x/y=w390:dbl)
                n98 = local write "Avg Scale - Last"(w391) -> ()
                n99 = local write "Avg Score - Last"(w390) -> ()
              }
            }
            "Avg Score" <- w149
            "Avg Scale" <- w84
            n100 = case shown="True" w85 {
              tunnel: w87 -> [w192 w196]
              tunnel: "5 / 4\nTransition Scale" -> [_ w195]
              tunnel: w84 -> [_ w194]
              tunnel: [w192 w193] -> w83
              frame False {
              }
              frame True {
                n101 = case shown="\"Sub - 2\", Default" w196 {
                  tunnel: w195 -> [w199 w205]
                  tunnel: w194 -> [w200 w206]
                  tunnel: [w197 w203] -> w193
                  frame "Sub - 2", Default {
                    n102 = Less Or Equal?(x=w200, y=w199) -> (x <= y?=w198:bool)
                    n103 = case shown="False" w198 {
                      tunnel: [T2."Sub - 2" ("Initial Template") T2."Normal - 5" ("Initial Template")] -> w197
                      frame False {
                      }
                      frame True {
                      }
                    }
                  }
                  frame "Normal - 5" {
                    n104 = Greater Or Equal?(x=w206, y=w205) -> (x >= y?=w204:bool)
                    n105 = case shown="True" w204 {
                      tunnel: [T2."Normal - 5" ("Initial Template") T2."Sub - 2" ("Initial Template")] -> w203
                      frame False {
                      }
                      frame True {
                      }
                    }
                  }
                }
              }
            }
            "Next Template" <- w83
            n106 = call "Scaling and Mapping"("Signals"=w84) -> ("Scaled Signals"=w152:dynamicdata)  [unwired: 9 in, 1 out]
            n107 = Unbundle By Name(w113) -> ("Minimum Match Score"=w120:sgl, "Range Settings"=w117:T5[])
            n108 = To Single Precision Float(number=w152) -> (single precision float=w151:sgl)
            "Scale \nCushion" <- w151
            n109 = Index Array(array=w117, index=u32 1) -> (element=w121:T5)
            n110 = Unbundle(w121) -> ("Min"=w119:dbl, "Max"=w118:dbl)  [unwired: 1 out]
            n111 = case shown="\"Normal - 5\"" w83 {
              tunnel: "ROI_factor(vertical) (5 b)" -> [_ _ w256]
              tunnel: "ROI_factor(Horiztonal) (5 b)" -> [_ _ w255]
              tunnel: "ROI_factor(vertical) (4 b)" -> [_ w253 _]
              tunnel: "ROI_factor(Horiztonal) (4 b)" -> [_ w252 _]
              tunnel: "ROI_factor(vertical) (2 b)" -> [w250 _ _]
              tunnel: "ROI_factor(Horiztonal) (2 b)" -> [w249 _ _]
              tunnel: [w250 w253 w256] -> w139
              tunnel: [w249 w252 w255] -> w138
              tunnel: "Minimum Score\nSub 2" -> [w248 _ _]
              tunnel: [w248 w251 w254] -> w137
              tunnel: "Minimum Score\nNormal 5" -> [_ _ w254]
              tunnel: "Minimum Score\nSub 4" -> [_ w251 _]
              frame "Sub - 2" {
              }
              frame "Sub - 4", Default {
              }
              frame "Normal - 5" {
              }
            }
            n112 = case shown="False" w153 {
              tunnel: w85 -> [w274 w387]
              tunnel: [FALSE w386] -> w107
              tunnel: w91 -> [w273 _]
              tunnel: w151 -> [w269 _]
              tunnel: "Score\nCushion" -> [w271 _]
              tunnel: w149 -> [w272 _]
              tunnel: w84 -> [w270 _]
              tunnel: w139 -> [w268 _]
              tunnel: w138 -> [w267 _]
              tunnel: w137 -> [w266 _]
              tunnel: w136 -> [w265 w385]
              tunnel: [w264 w383] -> w125
              tunnel: [w263 w379] -> w124
              tunnel: [w262 w378] -> w123
              tunnel: [w261 w385] -> w95
              tunnel: w120 -> [w260 _]
              tunnel: w119 -> [w259 _]
              tunnel: w118 -> [w258 _]
              frame False {
                n113 = case shown="True" w274 {
                  tunnel: w273 -> [_ w316]
                  tunnel: w272 -> [_ w315]
                  tunnel: w271 -> [_ w314]
                  tunnel: w270 -> [_ w313]
                  tunnel: w269 -> [_ w312]
                  tunnel: w268 -> [_ w311]
                  tunnel: w267 -> [_ w310]
                  tunnel: w266 -> [_ w302]
                  tunnel: [w278 w304] -> w261
                  tunnel: [w277 w301] -> w264
                  tunnel: [w276 w300] -> w263
                  tunnel: [w275 w299] -> w262
                  tunnel: w265 -> [_ w298]
                  tunnel: w260 -> [_ w297]
                  tunnel: w259 -> [_ w296]
                  tunnel: w258 -> [_ w295]
                  frame False {
                    # "Upper Scale"
                    # "Lower Scale"
                    # "Min Score"
                    # "Initial ROI Descriptor"
                    # "Check Lock Status of OTHER Cam,\n\nif True,\n\nthen use it's settings,\n\notherwise use default no lock"
                    n114 = shared-variable "RT myRIO Target - Overlord\\Localization_Variables_r0.lvlib\\Image Lock - R"() -> (w285:bool)  [unwired: 1 in, 1 out]
                    n115 = case shown="False" w285 {
                      tunnel: [w288 w292] -> w277
                      tunnel: [w286 w291] -> w275
                      tunnel: [w287 w290] -> w276
                      frame False {
                        n116 = Unbundle By Name("Default No Lock\nSetting Values") -> ("Min Score"=w288:dbl, "Min Scale"=w287:dbl, "Max Scale"=w286:dbl)
                      }
                      frame True {
                        n117 = shared-variable "RT myRIO Target - Overlord\\Localization_Variables_r0.lvlib\\Info - Right"() -> (w294:T3)  [unwired: 1 in, 1 out]
                        n118 = Unbundle(w294) -> ("Setting Values"=w293:T1)  [unwired: 3 out]
                        n119 = Unbundle(w293) -> ("Min Scale"=w290:dbl, "Max Scale"=w291:dbl, "Min Score"=w292:dbl)
                      }
                    }
                    n120 = Bundle(0, 0, 640, 480, 0) -> (w279:cluster{i32, i32, i32, i32, i32})  [unwired: 1 in]
                    n121 = call "IMAQ Convert Rectangle to ROI"("Rectangle"=w279) -> ("ROI Descriptor"=w278:T9)  [unwired: 8 in, 1 out]
                  }
                  frame True {
                    # "Apply Limit to Score"
                    # "Score out"
                    # "Apply Limits to ROI"
                    n122 = case shown="True" w316 {
                      tunnel: w315 -> [_ w362]
                      tunnel: w314 -> [_ w361]
                      tunnel: w313 -> [w336 w348]
                      tunnel: w312 -> [w343 w360]
                      tunnel: w311 -> [_ w355]
                      tunnel: w310 -> [_ w354]
                      tunnel: [w323 w351] -> w308
                      tunnel: [w322 w347] -> w307
                      tunnel: [w321 w350] -> w306
                      tunnel: [w320 w349] -> w305
                      tunnel: [w339 w346] -> w303
                      tunnel: [w338 w345] -> w300
                      tunnel: [w337 w344] -> w299
                      tunnel: w298 -> [w333 _]
                      tunnel: w297 -> [w319 _]
                      tunnel: w296 -> [w318 _]
                      tunnel: w295 -> [w317 _]
                      frame False {
                        # "Current Match was Invalid"
                        n123 = Divide(x=w343, y=sgl 3.0) -> (x/y=w341:sgl)
                        n124 = Subtract(x=w318, y=w341) -> (x-y=w338:dbl)
                        n125 = Add(x=w317, y=w341) -> (x+y=w337:dbl)
                        n126 = call "Scaling and Mapping2"("Signals"=w336) -> ("Scaled Signals"=w335:dynamicdata)  [unwired: 9 in, 1 out]
                        n127 = To Single Precision Float(number=w335) -> (single precision float=w328:sgl)
                        n128 = Subtract(x=w319, y="Score Decay \nFactor") -> (x-y=w339:dbl)
                        n129 = call "IMAQ Convert ROI to Rectangle"("ROI Descriptor"=w333) -> ("Rectangle"=w334:T13)  [unwired: 8 in, 1 out]
                        n130 = Unbundle By Name(w334) -> ("Left"=w327:i32, "Top"=w326:i32, "Right"=w325:i32, "Bottom"=w324:i32)
                        n131 = To Long Integer(number=w328) -> (32bit integer=w330:i32)
                        n132 = Divide(x=w328, y=sgl 10.0) -> (x/y=w332:sgl)
                        n133 = Subtract(x=w327, y=w330) -> (x-y=w323:i32)
                        n134 = Add(x=w325, y=w330) -> (x+y=w321:i32)
                        n135 = To Long Integer(number=w332) -> (32bit integer=w329:i32)
                        n136 = Subtract(x=w326, y=w329) -> (x-y=w322:i32)
                        n137 = Add(x=w324, y=w329) -> (x+y=w320:i32)
                      }
                      frame True {
                        w352 = sgl 109.0 ("x")
                        w353 = sgl 159.0 ("x")
                        # "Current Match was Valid"
                        # "Center of Image"
                        # "Main ROI"
                        # "Horizontal Scale \n(smaller number = smaller ROI)"
                        n138 = Subtract(x=w362, y=w361) -> (x-y=w346:dbl)
                        n139 = case shown="0, Default" "ROBOT STATE\n(fwd, bwd, neither)" {
                          tunnel: w348 -> [w367 w372 w377]
                          tunnel: [w366 w368 w373] -> w344
                          tunnel: w360 -> [w364 w371 w376]
                          tunnel: [w365 w369 w374] -> w345
                          frame 0, Default {
                            n140 = Subtract(x=w367, y=w364) -> (x-y=w365:dbl)
                            n141 = Add(x=w364, y=w367) -> (x+y=w366:dbl)
                          }
                          frame 1 {
                            n142 = Subtract(x=w372, y=5.0) -> (x-y=w369:dbl)
                            n143 = Add(x=w371, y=w372) -> (x+y=w368:dbl)
                          }
                          frame -1 {
                            n144 = Subtract(x=w377, y=w376) -> (x-y=w374:dbl)
                            n145 = Add(x=5.0 ("y"), y=w377) -> (x+y=w373:dbl)
                          }
                        }
                        n146 = Divide(x=w348, y=w355) -> (x/y=w358:dbl)
                        n147 = Multiply(x=w348, y=w354) -> (x*y=w356:dbl)
                        n148 = Divide(x=w356, y=sgl 2.0) -> (x/y=w359:dbl)
                        n149 = Add(x=w352, y=w358) -> (x+y=w349:dbl)
                        n150 = Subtract(x=w352, y=w358) -> (x-y=w347:dbl)
                        n151 = Subtract(x=w353, y=w359) -> (x-y=w351:dbl)
                        n152 = Add(x=w359, y=w353) -> (x+y=w350:dbl)
                      }
                    }
                    n153 = Greater?(x=w303, y=w302) -> (0:w309:bool)
                    n154 = call "Bound_RO_R_R0I.vi"("Bottom Right - Y"=w305, "Right - X"=w306, "Top Left - Y"=w307, "Top  Left - x"=w308) -> ("ROI Descriptor"=w304:T9)  [unwired: 7 in]
                    n155 = Select(t=w303, s=w309, f=w302) -> (s? t:f=w301:dbl)
                  }
                }
              }
              frame True {
                # "Pull Down Startup IF Already True and Lock\nOtherwise don't update"
                # "Still In Start - up, don't change anything"
                n156 = Not(x=w387) -> (.not. x?=w386:bool)
                n157 = local read "INITIAL Search Settings"() -> (w384:T6)
                n158 = Unbundle(w384) -> ("Range Settings"=w381:T5[], "Minimum Match Score"=w383:sgl)  [unwired: 5 out]
                n159 = Index Array(array=w381, index=1) -> (element=w380:T5)
                n160 = Unbundle(w380) -> ("Min"=w379:dbl, "Max"=w378:dbl)  [unwired: 1 out]
              }
            }
            n161 = call "IMAQ Overlay ROI"("ROI Descriptor"=w95, "Image"=w111) -> ("Image Out"=→"Right Image out":T7)  [unwired: 8 in, 1 out]
            n162 = Less?(x=w125, y="Absolute\nMinimum Score") -> (x < y?=w129:bool)
            n163 = Less?(x=w124, y="Absolute\nMinimum Scale") -> (x < y?=w132:bool)
            n164 = Greater?(x=w123, y="Absolute\nMaximum Scale") -> (0:w135:bool)
            n165 = Greater?(x=w124, y=w123) -> (0:w131:bool)
            n166 = Less?(x=w123, y=w124) -> (x < y?=w134:bool)
            n167 = Select(t="Absolute\nMinimum Score", s=w129, f=w125) -> (s? t:f=w106:dbl)
            "New Min Score" <- w106
            n168 = Or(x=w132, y=w131) -> (x .or. y?=w130:bool)
            n169 = Or(x=w135, y=w134) -> (x .or. y?=w133:bool)
            n170 = Select(t="Absolute\nMinimum Scale", s=w130, f=w124) -> (s? t:f=w105:dbl)
            "New Low Scale" <- w105
            n171 = Select(t="Absolute\nMaximum Scale", s=w133, f=w123) -> (s? t:f=w104:dbl)
            "New high Scale" <- w104
            n172 = Bundle("index"=w116, "Min"=w105, "Max"=w104) -> (w115:cluster{"index":u32, "Min":dbl, "Max":dbl})  [unwired: 1 in]
            n173 = Replace Array Subset(array=w117, new element=w115, index=w116) -> (w114:T5[])
            n174 = Bundle By Name(cluster=w113, "Minimum Match Score"=w106, "Range Settings"=w114) -> (w112:T6)
            n175 = local read "Current Template"() -> (w109:T2)
            n176 = local read "Next Template"() -> (w94:T2)
            n177 = Equal?(x=w109, y=w94) -> (x = y?=w110:bool)
            n178 = Bundle("Minimum Score\nNormal 5"=w106, "Min"=w105, "Max"=w104) -> (w103:T14)  [unwired: 1 in]
            n179 = case shown="False" w110 {
              tunnel: w109 -> [_ w245]
              tunnel: w108 -> [w217 w247]
              tunnel: w91 -> [w210 w246]
              tunnel: [w209 w244] -> w102
              tunnel: w100 -> [w218 _]
              tunnel: w103 -> [w213 w243]
              tunnel: w94 -> [w211 _]
              frame False {
                # "Check if Tracking is Available for the Next Template State"
                n180 = case shown="\"Normal - 5\"" w211 {
                  tunnel: [0 1 2 1] -> w216
                  frame "Sub - 2", Default {
                  }
                  frame "Sub - 3" {
                  }
                  frame "Sub - 4" {
                  }
                  frame "Normal - 5" {
                  }
                }
                n181 = Index Array(array=w218, index=w216) -> (element=w219:bool)
                n182 = local read "Y Coordinates"() -> (w214:sgl[])
                n183 = local read "X Coordinates"() -> (w215:sgl[])
                n184 = case shown="True" w219 {
                  tunnel: w215 -> [_ w238]
                  tunnel: w214 -> [_ w237]
                  tunnel: [w220 w234] -> w212
                  tunnel: w217 -> [w220 w235]
                  tunnel: w216 -> [_ w236]
                  frame False {
                  }
                  frame True {
                    w231 = sgl 0.4 ("y")
                    n185 = Unbundle(w235) -> ("x"=w232:dbl, "y"=w230:dbl)
                    n186 = Index Array(array=w238, index=w236) -> (element=w227:sgl)
                    n187 = Index Array(array=w237, index=w236) -> (element=w228:sgl)
                    n188 = Subtract(x=sgl 1.0, y=w231) -> (x-y=w229:sgl)
                    n189 = Multiply(x=w229, y=w227) -> (x*y=w225:sgl)
                    n190 = Multiply(x=w229, y=w228) -> (x*y=w223:sgl)
                    n191 = Multiply(x=w231, y=w232) -> (x*y=w226:dbl)
                    n192 = Multiply(x=w231, y=w230) -> (x*y=w224:dbl)
                    n193 = Add(x=w226, y=w225) -> (x+y=w222:dbl)
                    n194 = Add(x=w224, y=w223) -> (x+y=w221:dbl)
                    n195 = Bundle(w222, w221) -> (w234:cluster{dbl, dbl})  [unwired: 1 in]
                  }
                }
                n196 = Bundle("Position"=w212, w210, "Next Template"=w211, w213) -> (w209:T15)  [unwired: 1 in]
              }
              frame True {
                n197 = Bundle("Position"=w247, w246, "Current Template"=w245, w243) -> (w244:T16)  [unwired: 1 in]
              }
            }
            "Tracking Info" <- w102
            n198 = shared-variable "RT myRIO Target - Overlord\\Localization_Variables_r0.lvlib\\Info - Left"(w102) -> ()  [unwired: 1 in, 1 out]
          }
          frame #2 {
            n199 = shared-variable "RT myRIO Target - Overlord\\Localization_Variables_r0.lvlib\\Left Servo Angle_Image"(w583) -> ()  [unwired: 1 in, 1 out]
            n200 = shared-variable "RT myRIO Target - Overlord\\Localization_Variables_r0.lvlib\\Left_Flag"(TRUE ("RIGHT_FLAG")) -> ()  [unwired: 1 in, 1 out]
          }
        }
        "Startup Flag" <- w64
        "Valid Scale History" <- w50
        "Valid Beacon History - in" <- w52
        "Valid Score History" <- w48
        "Current Search Settings" <- w66
        "Current Template" <- w74
      }
    }
  }
